vi "Simple Timer.vi"(7 "Case Select":enum16{"Get Time", "Initialize"}(ring), 8 "Error in":errorcluster) -> (0 "error out":errorcluster, 2 "Time Elapsed?":bool=TRUE, 3 "Elapsed Time":dbl)   [LabVIEW 2023, in "Internal Communication.lvlib"]
uses:
  Project-Based-Learning/Internal Communication/Internal Communication.lvlib
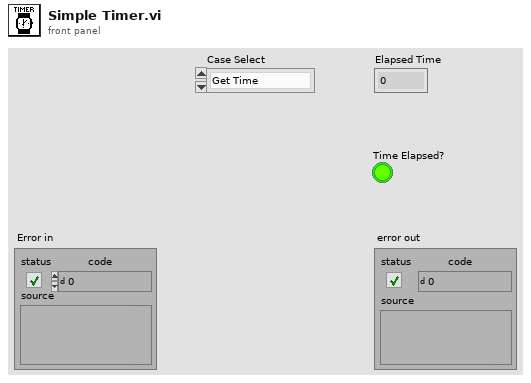
[diagram p1: front panel]
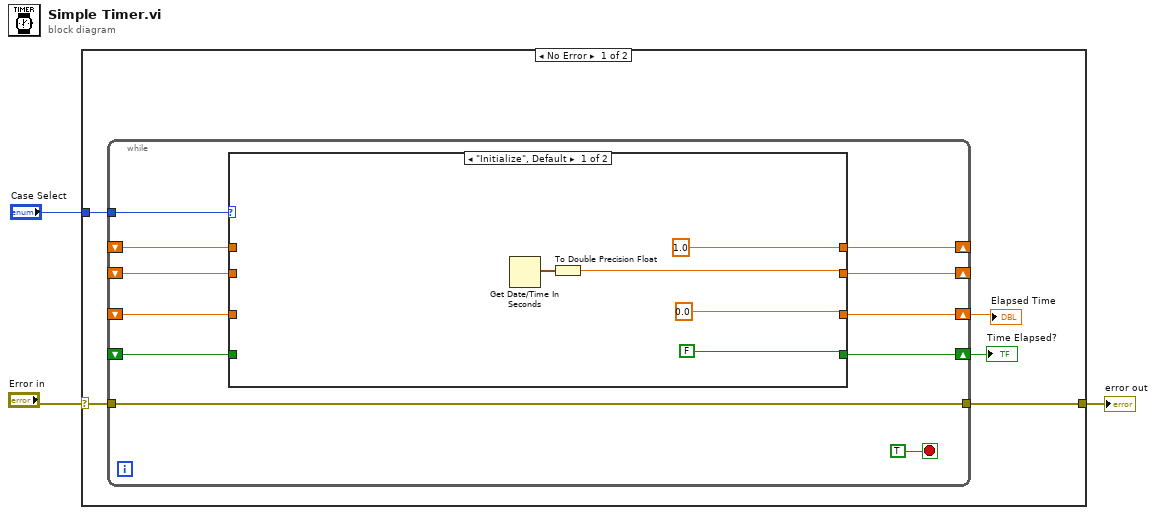
[diagram p0: block diagram]
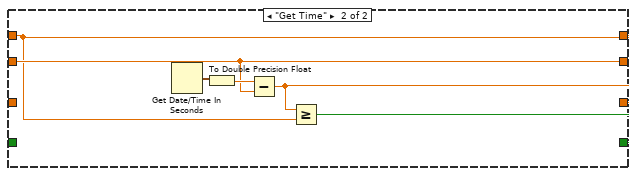
[diagram p2: hidden frame]
diagram:
  n1 = case shown="No Error" "Error in" {
    selector: "Error in" -> [w5 w31]
    tunnel: [w4 w31] -> w2
    tunnel: "Case Select" -> [w8 _]
    frame No Error {
      n2 = while {
        tunnel: w8 -> [w18]
        shift-right: [w16] -> _
        shift-left: _ -> [w17]
        shift-right: [w15] -> w7
        shift-left: _ -> [w14]
        shift-right: [w13] -> w6
        shift-left: _ -> [w12]
        shift-right: [w11] -> _
        shift-left: _ -> [w10]
        tunnel: w5 -> [w9]
        tunnel: [w9] -> w4
        stop <- TRUE stop-if-true
        n3 = case shown="\"Initialize\", Default" w18 {
          tunnel: w17 -> [_ w25]
          tunnel: [1.0 ("Target Time") w25] -> w16
          tunnel: [0.0 ("Elapsed Time") w28] -> w15
          tunnel: w14 -> [_ _]
          tunnel: [FALSE ("Time Elapsed?") w27] -> w13
          tunnel: w12 -> [_ _]
          tunnel: [w21 w26] -> w11
          tunnel: w10 -> [_ w26]
          frame "Initialize", Default {
            n4 = Get Date/Time In Seconds() -> (seconds since 1Jan1904=w22:timestamp)
            n5 = To Double Precision Float(number=w22) -> (double precision float=w21:dbl)
          }
          frame "Get Time" {
            n6 = Get Date/Time In Seconds() -> (seconds since 1Jan1904=w30:timestamp)
            n7 = To Double Precision Float(number=w30) -> (double precision float=w29:dbl)
            n8 = Subtract(x=w29, y=w26) -> (x-y=w28:dbl)
            n9 = Greater Or Equal?(x=w28, y=w25) -> (x >= y?=w27:bool)
          }
        }
      }
      "Elapsed Time" <- w7
      "Time Elapsed?" <- w6
    }
    frame Error {
      # "Case structure checks for errors - if there's an errorr, do nothing except pass the error back out"
    }
  }
  "error out" <- w2
